vi "HW Initialize.vi"(8 "Simulate Failure":bool, 10 "ECU":string, 11 "Socket":u32) -> (0 "error out":errorcluster, 1 "Connection Ref":refnum<k5>, 2 "Report Text":string, 3 "Test Result":bool)   [LabVIEW 2024, in "Shared Steps.lvlib"]
doc: "Connect to ECU"
uses:
  Shared Steps.lvlib
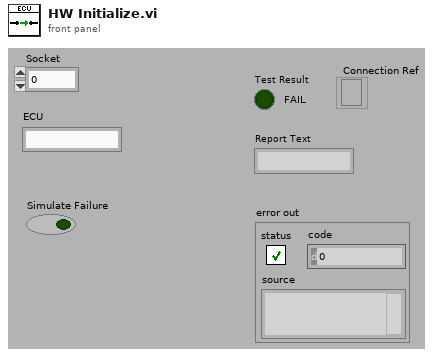
[diagram p1: front panel]
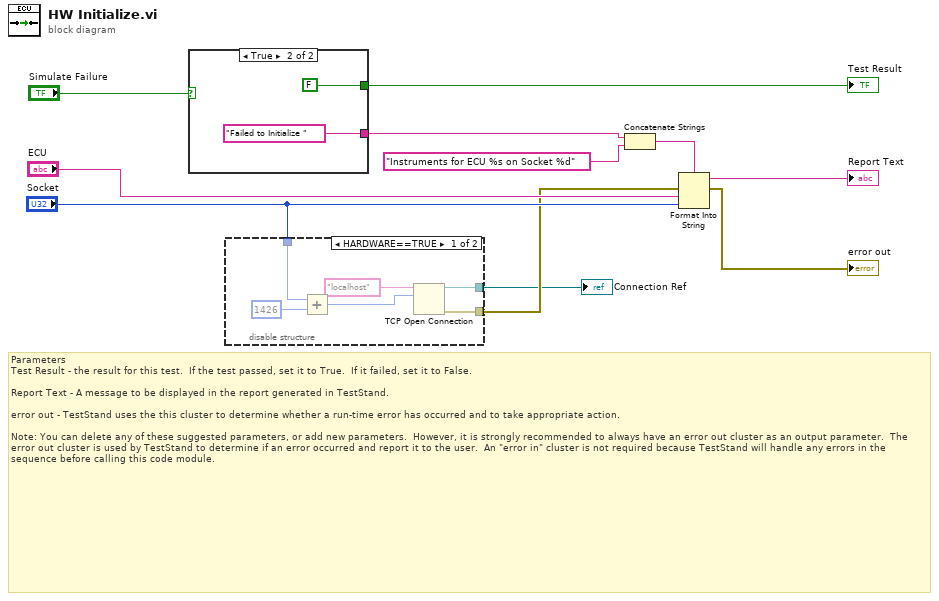
[diagram p0: block diagram]
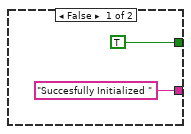
[diagram p3: hidden frame]
diagram:
  # "Parameters\nTest Result - the result for this test.  If the test passed, set it to True.  If it failed, set it to False. \n\nReport Text - A message to be displayed in the report generated in TestStand. \n\nerror out - TestStand uses the this cluster to determine whether a run-time error has occurred and to take appropriate action.  \n\nNote: You can delete any of these suggested parameters, or add new parameters.  However, it is strongly recommended to always have an error out cluster as an output parameter.  The error out cluster is used by TestStand to determine if an error occurred and report it to the user.  An \"error in\" cluster is not required because TestStand will handle any errors in the sequence before calling this code module."
  n1 = case shown="True" "Simulate Failure" {
    tunnel: ["Succesfully Initialized " "Failed to Initialize "] -> w5
    tunnel: [TRUE FALSE] -> w4
    frame False {
    }
    frame True {
    }
  }
  "Test Result" <- w4
  n2 = disable-structure shown="HARDWARE==TRUE" {
    disable-tunnel: "Socket" -> [w20 _]
    disable-tunnel: [w19 _] -> w2
    disable-tunnel: [w16 _] -> w1
    frame condition #0 {
      n3 = Add(x=w20, y=u16 1426 ("remote port or service name")) -> (x+y=w17:u32)
      n4 = TCP Open Connection(address="localhost", remote port or service name=w17) -> (connection ID=w16:refnum<k5>, error out=w19:errorcluster)  [unwired: 3 in]
    }
    frame condition #1 (active) {
    }
  }
  "Connection Ref" <- w1
  n5 = Concatenate Strings(w5, "Instruments for ECU %s on Socket %d" ("format string")) -> (w7:string)
  n6 = Format Into String(format string=w7, error in=w2, "ECU", "Socket") -> (resulting string=→"Report Text":string, error out=→"error out":errorcluster)  [unwired: 1 in]
